vi "Configure Advanced PID Parameters.vi"(6 "Manual Reset (0)":i32, 7 "Unit Address (1)":u8=1, 8 "error in (no error)":errorcluster, 9 "Relative Cool/Ch2 Gain (0)":i32, 10 "PID Number  (1)":u8=1 min=1 max=3, 11 "VISA resource name":refnum<visa-resource-name>) -> (0 "error out":errorcluster, 3 "VISA resource name out":refnum<visa-resource-name>)   [LabVIEW 2014, in "Eurotherm 35xx Series.lvlib"]
doc: "This VI sets advanced PID parameters."
uses:
  <instrlib>/Eurotherm 35xx Series/Eurotherm 35xx Series.lvlib
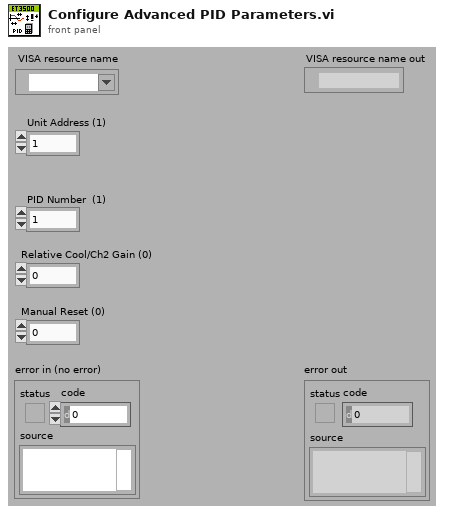
[diagram p1: front panel]
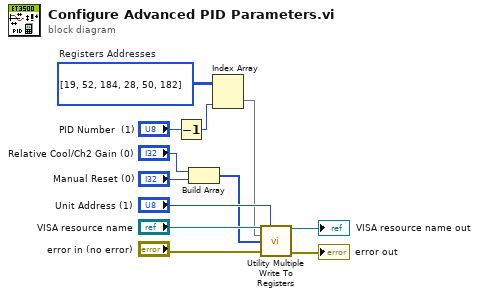
[diagram p0: block diagram]
diagram:
  w12 = u16[][] [[19, 52, 184], [28, 50, 182]]  # Registers Addresses
  n1 = Decrement(x="PID Number  (1)") -> (x-1=w10:u8)
  n2 = Build Array("Relative Cool/Ch2 Gain (0)", "Manual Reset (0)") -> (w1:i32[])
  n3 = Index Array(array=w12, index (col)=w10) -> (element=w2:u16[])  [unwired: 1 in]
  n4 = call <instrlib>:"Utility Multiple Write To Registers.vi"("VISA resource name"="VISA resource name", "Unit Address (1)"="Unit Address (1)", "Registers Addresses (0)"=w2, "Data (0)"=w1, "error in (no error)"="error in (no error)") -> ("VISA resource name out"=→"VISA resource name out":refnum<visa-resource-name>, "error out"=→"error out":errorcluster)  [unwired: 9 in]
